vi "AppendLine seperator.vi"(0 "PDF Report IN":refnum<class "PDF Report Class.lvclass">, 2 "H/F Line":T1={"H/F Line"=enum."Horizontal line", "Thickness (point)"=0.75, " Colour"=7171459}, 11 "error in (no error)":errorcluster, 13 "Position":T3) -> (4 "PDF Report OUT":refnum<class "PDF Report Class.lvclass">, 15 "error out":errorcluster)   [LabVIEW 2019]
doc: "Appends a <B>horizontal line</B> to separate the header (or footer) of the page.\n\n<B>FRANÇAIS</B>\nAjoute une <B>ligne horizontale</B> qui sépare l'en-tête ou le pied de page du texte du rapport.\n\n\n\nVersion 1.0\nDeveloped by Jean-Marc Simard\nCopyright © 2010, Exaprom Inc.\nAll rights reserved.\nLicense: BSD\n\nWith iTextSharp 4.1.6 (http://itextsharp.sourceforge.net)\nunder Mozilla Public License Version 1.1\n(http://www.mozilla.org/MPL/MPL-1.1.html)"
uses:
  <userlib>/Exaprom PDF/LV Class/PDF Report Class/PDF Report Class.lvclass
  <userlib>/Exaprom PDF/Controls/Header, Footer and Watermark Controls/Header or Footer.ctl
  <userlib>/Exaprom PDF/Controls/Header, Footer and Watermark Controls/Header or Footer Line cluster.ctl
  <userlib>/Exaprom PDF/Controls/Header, Footer and Watermark Controls/Header Footer Line.ctl
  C:/Program Files/National Instruments/LabVIEW 2019/user.lib/Exaprom PDF/DLL/itextsharp.dll
  DLL/itextsharp.dll
  <userlib>/Exaprom PDF/LV Class/Header and Footer Class/Header and Footer Class.lvclass
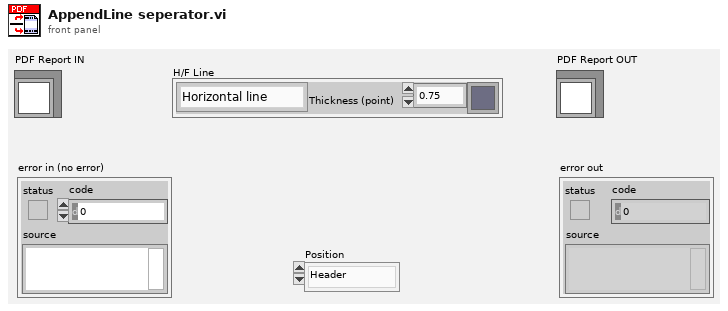
[diagram p1: front panel]
types:
  T1 = typedef "Header or Footer Line cluster.ctl" = cluster{"H/F Line":T2, "Thickness (point)":sgl, " Colour":u32}
  T2 = typedef "Header Footer Line.ctl" = enum16{"No line", "Horizontal line"}
  T3 = typedef "Header or Footer.ctl" = enum16{"Header", "Footer"}
  T4 = typedef "Header Footer [ ] V2.ctl" = T5[]
  T5 = typedef "Header Footer cluster V2.ctl" = cluster{"Header or Footer":T3, "Start page":i32, "Start with #":i32, "Type":T6, "Alignment":T7, "Vertical Alignement":T8, "Line spacing":T9, "Image (%)":sgl, "Page #":T10, "Text":string, "Path":string, "Font":T11, "Font refnum":refnum<k24>, "Line":cluster{"Line":T2, "Thickness (points)":sgl, "Colour":T13}, "Vert margin":dbl, "Hyperlink":string}
  T6 = typedef "Header Footer Type.ctl" = enum16{"Select", "Text", "Text + hyperlink", "Page number", "Image", "Image + hyperlink"}
  T7 = typedef "Header footer horiz alignment.ctl" = enum16{"Left", "Center", "Right"}
  T8 = typedef "Cell Vertical alignment.ctl" = enum16{"TOP", "MIDDLE", "BOTTOM"}
  T9 = typedef "Line spacing.ctl" = enum16{"Select", "1.0", "1.5", "2.0"}
  T10 = typedef "Page number.ctl" = cluster{"Text 1":string, "Text 2":string, "Text 3":string}
  T11 = typedef "Font complete cluster horizontal.ctl" = cluster{"Name":string, "Size":T12, "Color":T13, "Style":cluster{"Bold":bool, "Italic":bool, "Underline":bool, "Strikeout":bool}, "Type":T14}
  T12 = typedef "Font size.ctl" = sgl
  T13 = typedef "Font color.ctl" = u32
  T14 = typedef "Type and encoding.ctl" = cluster{"Type&direction":T15, "Embedded":bool, "Encoding":string}
  T15 = typedef "Type and run direction.ctl" = enum16{"Select", "ASCII", "UTF-16", "UTF-16 (default)", "UTF-16 (LTR)", "UTF-16 (RTL)"}
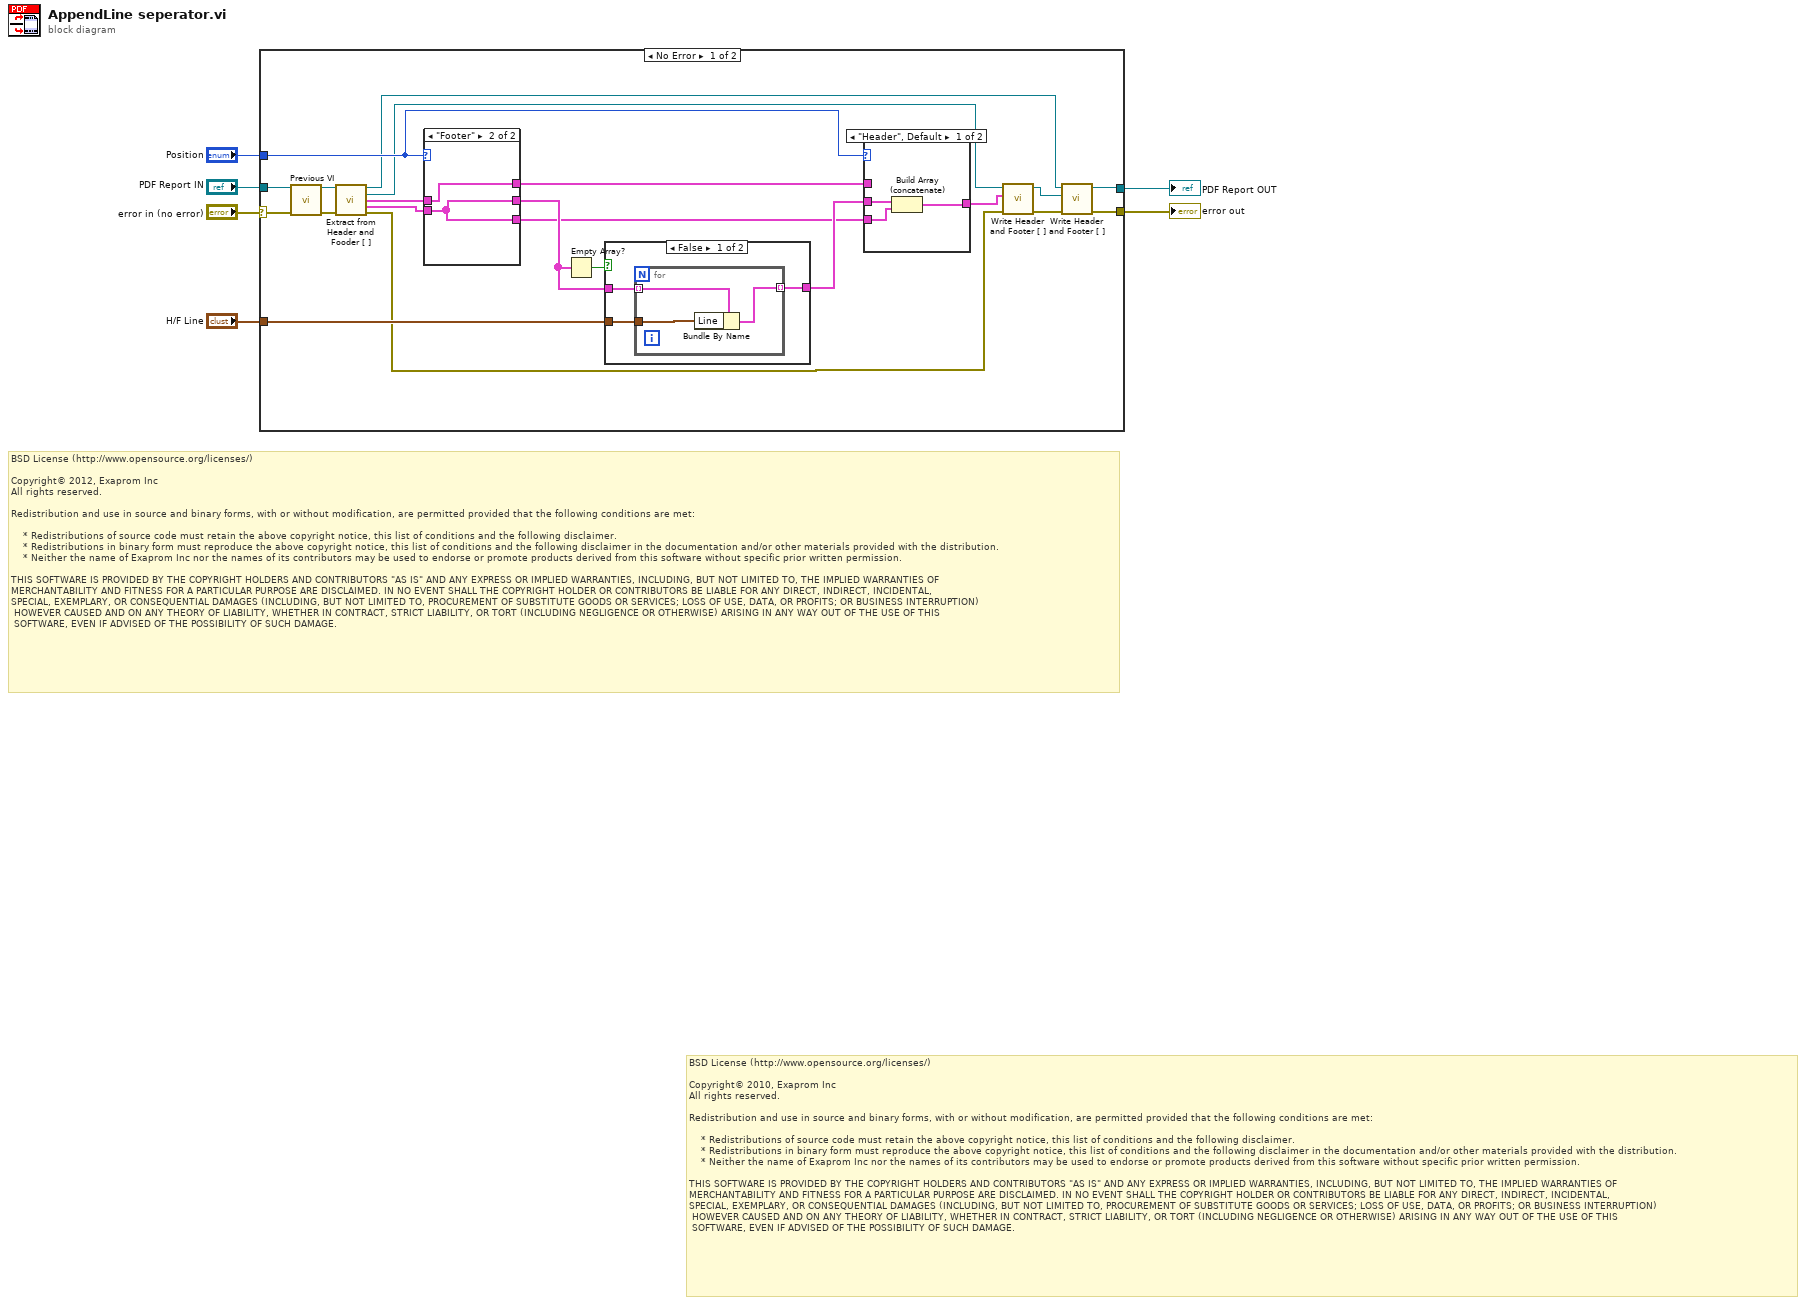
[diagram p0: block diagram]
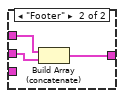
[diagram p4: hidden frame]
diagram:
  # "BSD License (http://www.opensource.org/licenses/)\n\nCopyright© 2012, Exaprom Inc\nAll rights reserved.\n\nRedistribution and use in source and binary forms, with or without modification, are permitted provided that the following conditions are met:\n\n    * Redistributions of source code must retain the above copyright notice, this list of conditions and the following disclaimer.\n    * Redistributions in binary form must reproduce the above copyright notice, this list of conditions and the following disclaimer in the documentation and/or other materials provided with the distribution.\n    * Neither the name of Exaprom Inc nor the names of its contributors may be used to endorse or promote products derived from this software without specific prior written permission.\n\nTHIS SOFTWARE IS PROVIDED BY THE COPYRIGHT HOLDERS AND CONTRIBUTORS \"AS IS\" AND ANY EXPRESS OR IMPLIED WARRANTIES, INCLUDING, BUT NOT LIMITED TO, THE IMPLIED WARRANTIES OF \nMERCHANTABILITY AND FITNESS FOR A PARTICULAR PURPOSE ARE DISCLAIMED. IN NO EVENT SHALL THE COPYRIGHT HOLDER OR CONTRIBUTORS BE LIABLE FOR ANY DIRECT, INDIRECT, INCIDENTAL,\nSPECIAL, EXEMPLARY, OR CONSEQUENTIAL DAMAGES (INCLUDING, BUT NOT LIMITED TO, PROCUREMENT OF SUBSTITUTE GOODS OR SERVICES; LOSS OF USE, DATA, OR PROFITS; OR BUSINESS INTERRUPTION)\n HOWEVER CAUSED AND ON ANY THEORY OF LIABILITY, WHETHER IN CONTRACT, STRICT LIABILITY, OR TORT (INCLUDING NEGLIGENCE OR OTHERWISE) ARISING IN ANY WAY OUT OF THE USE OF THIS\n SOFTWARE, EVEN IF ADVISED OF THE POSSIBILITY OF SUCH DAMAGE."
  # "BSD License (http://www.opensource.org/licenses/)\n\nCopyright© 2010, Exaprom Inc\nAll rights reserved.\n\nRedistribution and use in source and binary forms, with or without modification, are permitted provided that the following conditions are met:\n\n    * Redistributions of source code must retain the above copyright notice, this list of conditions and the following disclaimer.\n    * Redistributions in binary form must reproduce the above copyright notice, this list of conditions and the following disclaimer in the documentation and/or other materials provided with the distribution.\n    * Neither the name of Exaprom Inc nor the names of its contributors may be used to endorse or promote products derived from this software without specific prior written permission.\n\nTHIS SOFTWARE IS PROVIDED BY THE COPYRIGHT HOLDERS AND CONTRIBUTORS \"AS IS\" AND ANY EXPRESS OR IMPLIED WARRANTIES, INCLUDING, BUT NOT LIMITED TO, THE IMPLIED WARRANTIES OF \nMERCHANTABILITY AND FITNESS FOR A PARTICULAR PURPOSE ARE DISCLAIMED. IN NO EVENT SHALL THE COPYRIGHT HOLDER OR CONTRIBUTORS BE LIABLE FOR ANY DIRECT, INDIRECT, INCIDENTAL,\nSPECIAL, EXEMPLARY, OR CONSEQUENTIAL DAMAGES (INCLUDING, BUT NOT LIMITED TO, PROCUREMENT OF SUBSTITUTE GOODS OR SERVICES; LOSS OF USE, DATA, OR PROFITS; OR BUSINESS INTERRUPTION)\n HOWEVER CAUSED AND ON ANY THEORY OF LIABILITY, WHETHER IN CONTRACT, STRICT LIABILITY, OR TORT (INCLUDING NEGLIGENCE OR OTHERWISE) ARISING IN ANY WAY OUT OF THE USE OF THIS\n SOFTWARE, EVEN IF ADVISED OF THE POSSIBILITY OF SUCH DAMAGE."
  n1 = case shown="No Error" "error in (no error)" {
    selector: "error in (no error)" -> [w24 w44]
    tunnel: "PDF Report IN" -> [w27 w45]
    tunnel: "Position" -> [w20 _]
    tunnel: [w8 w45] -> w4
    tunnel: "H/F Line" -> [w23 _]
    tunnel: [w9 w44] -> w1
    frame No Error {
      n2 = call <userlib>:"Previous VI.vi"("PDF Report IN"=w27, "error in (no error)"=w24) -> ("PDF Report OUT"=w22:refnum<class "PDF Report Class.lvclass">, "error out"=w21:errorcluster)  [unwired: 12 out]
      n3 = call <userlib>:"Extract from Header and Fooder [ ].vi"("PDF Report IN"=w22, "error in (no error)"=w21) -> ("PDF Report OUT"=w7:refnum<class "PDF Report Class.lvclass">, "Header and Footer duplicate"=w14:refnum<class "Header and Footer Class.lvclass">, "Header [ ]"=w19:T4, "Footer [ ]"=w18:T4, "error out"=w12:errorcluster)  [unwired: 9 in]
      n4 = case shown="\"Footer\"" w20 {
        tunnel: w19 -> [w28 w30]
        tunnel: [w28 w29] -> w17
        tunnel: w18 -> [_ w29]
        tunnel: [_ w30] -> w16
        tunnel: [_ w29] -> w15
        frame "Header", Default {
        }
        frame "Footer" {
        }
      }
      n5 = Empty Array?(array=w17) -> (empty?=w25:bool)
      n6 = case shown="False" w25 {
        tunnel: w23 -> [w33 _]
        tunnel: w17 -> [w32 w37]
        tunnel: [w31 w37] -> w26
        frame False {
          n7 = for {
            tunnel: w33 -> [w36]
            tunnel: w32 -> [w35] mode=indexing
            tunnel: [w34] -> w31 mode=indexing
            n8 = Bundle By Name(cluster=w35, "Line"=w36) -> (w34:T5)
          }
        }
        frame True {
        }
      }
      n9 = case shown="\"Header\", Default" w20 {
        tunnel: w26 -> [w40 w42]
        tunnel: w16 -> [_ w43]
        tunnel: w15 -> [w39 _]
        tunnel: [w38 w41] -> w13
        frame "Header", Default {
          n10 = Build Array (concatenate)(w40, w39) -> (w38:T4)
        }
        frame "Footer" {
          n11 = Build Array (concatenate)(w43, w42) -> (w41:T4)
        }
      }
      n12 = call-dynamic "Write Header and Footer [ ].vi"("error in (no error)"=w12, "Header and Footer [ ]"=w13, "Header and Footer Class in"=w14) -> ("error out"=w10:errorcluster, "Header and Footer Class out"=w11:refnum<class "Header and Footer Class.lvclass">)  [unwired: 7 in]
      n13 = call-dynamic "Write Header and Footer [ ].vi"("error in (no error)"=w10, "Header and Footer Class.lvclass"=w11, "PDF Report Class in"=w7) -> ("error out"=w9:errorcluster, "PDF Report Class out"=w8:refnum<class "PDF Report Class.lvclass">)  [unwired: 7 in]
    }
    frame Error {
    }
  }
  "PDF Report OUT" <- w4
  "error out" <- w1
